vi "DeleteMission.vi"(6 "OldVal":bool, 7 "ID# To Delete (miss)":u16, 8 "error in (no error)":errorcluster, 10 "Initialized Mission Arrays in":T1 {"Readable Missions"."Points of Interest"."North" format="%#_10f"; "Readable Missions"."Points of Interest"."East" format="%#_8f"}, 11 "NetworkStreamWriter in":refnum<class "NetworkStreamWriter.lvclass">) -> (0 "error out":errorcluster, 2 "Initialized Mission Arrays out":T1 {"Readable Missions"."Points of Interest"."North" format="%#_10f"; "Readable Missions"."Points of Interest"."East" format="%#_8f"}, 3 "NetworkStreamWriter out":refnum<class "NetworkStreamWriter.lvclass">)   [LabVIEW 2013]
doc: "This VI takes the \"ID to Delete\" value and\n1) Sends that ID down to the forebrain\n2) Deletes the objects with that ID from the OCU mission arrays\n\nEric Schneider, August 2014"
uses:
  TypeDef/mission_arrays.ctl
  cRIO_Code/Data/TypeDefs/MissionDescription.ctl
  cRIO_Code/Data/TypeDefs/MissionTypeControl.ctl
  cRIO_Code/Data/TypeDefs/UTM Location.ctl
  cRIO_Code/Logic/Classes/Missions/GenericMission/GenericMission.lvclass
  RIO-OCU_Comm/NetworkStreams/Writer/NetworkStreamWriter.lvclass
  CommandMessages.ctl
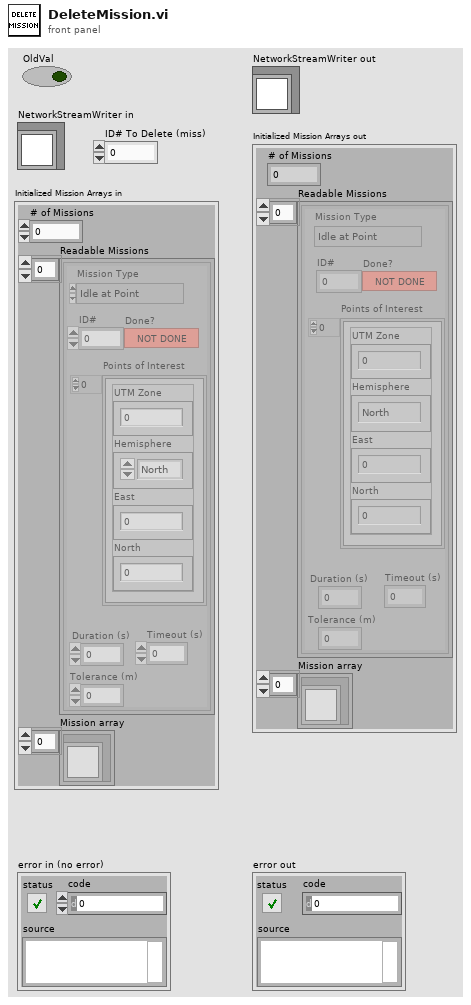
[diagram p1: front panel]
types:
  T1 = typedef "mission_arrays.ctl" = cluster{"# of Missions":i32, "Readable Missions":T2[], "Mission array":refnum<class "GenericMission.lvclass">[]}
  T2 = typedef "MissionDescription.ctl" = cluster{"Duration (s)":dbl, "Timeout (s)":dbl, "Tolerance (m)":dbl, "Mission Type":T3, "Points of Interest":T4[], "ID#":i32, "Done?":bool}
  T3 = typedef "MissionTypeControl.ctl" = enum16{"Idle at Point", "Drive to Waypoint", "Round Buoy to Port", "Round Buoy to Starboard", "Pass Between Buoys", "Station Keeping"}
  T4 = typedef "UTM Location.ctl" = cluster{"UTM Zone":dbl, "Hemisphere":enum16{"North", "South"}, "East":dbl, "North":dbl}
  T5 = typedef "CommandMessages.ctl" = enum16{"Pass", "OverrideMode", "Add mission", "Delete mission", "Add obstacle", "Delete obstacle", "Change constants"}
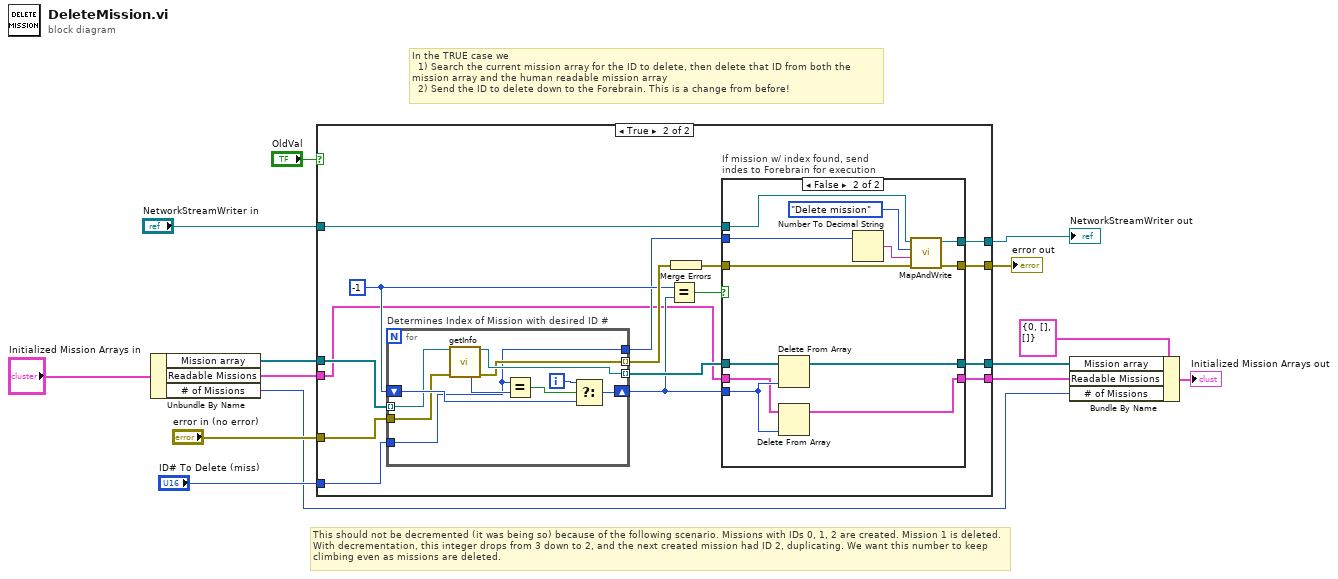
[diagram p0: block diagram]
diagram:
  # "This should not be decremented (it was being so) because of the following scenario. Missions with IDs 0, 1, 2 are created. Mission 1 is deleted. With decrementation, this integer drops from 3 down to 2, and the next created mission had ID 2, duplicating. We want this number to keep climbing even as missions are deleted."
  # "In the TRUE case we\n  1) Search the current mission array for the ID to delete, then delete that ID from both the mission array and the human readable mission array\n  2) Send the ID to delete down to the Forebrain. This is a change from before!"
  n1 = Unbundle By Name("Initialized Mission Arrays in") -> ("Mission array"=w8:refnum<class "GenericMission.lvclass">[], "Readable Missions"=w9:T2[], "# of Missions"=w1:i32)
  n2 = case shown="True" "OldVal" {
    tunnel: w8 -> [w15 w34]
    tunnel: [w15 w30] -> w12
    tunnel: [w16 w32] -> w13
    tunnel: [w17 w29] -> w3
    tunnel: "error in (no error)" -> [w17 w31]
    tunnel: "NetworkStreamWriter in" -> [w18 w24]
    tunnel: [w18 w28] -> w6
    tunnel: w9 -> [w16 w20]
    tunnel: "ID# To Delete (miss)" -> [_ w19]
    frame False {
    }
    frame True {
      w22 = -1
      n3 = for "Determines Index of Mission with desired ID #" {
        tunnel: w34 -> [w52] mode=indexing
        tunnel: [w60] -> w33 mode=indexing
        shift-right: [w57] -> w23
        shift-left: w22 -> [w56]
        tunnel: [w55] -> w26 mode=indexing
        tunnel: w31 -> [w54]
        tunnel: [w51] -> w21
        tunnel: w19 -> [w51]
        i -> [w58]
        n4 = call-dynamic "getInfo.vi"("GenericMission in"=w52, "error in (no error)"=w54) -> ("GenericMission out"=w60:refnum<class "GenericMission.lvclass">, "ID#"=w53:i16, "error out"=w55:errorcluster)  [unwired: 5 in, 6 out]
        n5 = Equal?(x=w51, y=w53) -> (x = y?=w59:bool)
        n6 = Select(t=w58, s=w59, f=w56) -> (s? t:f=w57:i32)
      }
      n7 = Equal?(x=w22, y=w23) -> (x = y?=w27:bool)
      n8 = Merge Errors(w26) -> (w25:errorcluster)
      n9 = case "If mission w/ index found, send\nindes to Forebrain for execution" shown="False" w27 {
        tunnel: w33 -> [w36 w50]
        tunnel: [w35 w49] -> w32
        tunnel: w23 -> [_ w48]
        tunnel: w24 -> [w37 w47]
        tunnel: w25 -> [w38 w41]
        tunnel: [w36 w44] -> w30
        tunnel: [w38 w42] -> w29
        tunnel: [w37 w43] -> w28
        tunnel: w21 -> [_ w40]
        tunnel: w20 -> [w35 w39]
        frame True {
        }
        frame False {
          n10 = Delete From Array(array=w50, index=w48) -> (array with subset deleted=w44:refnum<class "GenericMission.lvclass">[])  [unwired: 1 in, 1 out]
          n11 = Delete From Array(array=w39, index=w48) -> (array with subset deleted=w49:T2[])  [unwired: 1 in, 1 out]
          n12 = Number To Decimal String(number=w40) -> (decimal integer string=w45:string)  [unwired: 1 in]
          n13 = call "MapAndWrite.vi"("error in (no error)"=w41, "String_Cast_of_Info"=w45, "Commands"=CommandMessages."Delete mission", "NetworkStreamWriter in"=w47) -> ("error out"=w42:errorcluster, "NetworkStreamWriter out"=w43:refnum<class "NetworkStreamWriter.lvclass">)  [unwired: 2 in]
        }
      }
    }
  }
  "NetworkStreamWriter out" <- w6
  "error out" <- w3
  n14 = Bundle By Name(cluster=T1 {"# of Missions"=0, "Readable Missions"=[], "Mission array"=[]} ("Initialized Mission Arrays"), "Mission array"=w12, "Readable Missions"=w13, "# of Missions"=w1) -> (→"Initialized Mission Arrays out":T1)
